vi "Kalman Calculation.vi"(4 "our_robots":bool=TRUE, 5 "u_k":T1, 6 "R":T1=[[0.1, 0.0, 0.0], [0.0, 0.1, 0.0], [0.0, 0.0, 0.1]], 7 "Use Observation":bool=TRUE, 8 "intervalo":dbl=1.0, 9 "Pk-1|k-1":T1, 10 "x_k-1|k-1":T1=[[0.0, 0.0, 0.0], [0.0, 0.0, 0.0], [0.0, 0.0, 0.0]], 11 "z_k":T1) -> (1 "Conf":dbl, 2 "Pk|k":T1, 3 "x_k|k":T1)   [LabVIEW 2017]
uses:
  <vilib>/Analysis/Matrix/Datatypes/RealMatrix.ctl
  <vilib>/Analysis/_algsub.llb/Real Matrix Norm.vi
  <vilib>/Analysis/Matrix/Numeric/Multiply/Multiply - RM,R.vi
  <vilib>/Analysis/Matrix/Numeric/Conversions/Array To Matrix - RA2.vi
  <vilib>/Analysis/Matrix/Numeric/Multiply/Multiply - RM,RM.vi
  <vilib>/Analysis/Matrix/Numeric/Add/Add - RM,RM.vi
  <vilib>/Analysis/baseanly.llb/Real Inverse Matrix.vi
  <vilib>/Analysis/Matrix/Numeric/Subtract/Subtract - RM,RM.vi
  <vilib>/Analysis/Matrix/NI_Matrix.lvlib
  <vilib>/Analysis/NI_AALBase.lvlib
  <vilib>/Analysis/NI_AALPro.lvlib
panel:
  out "In Range?":bool[][](array[boolean])
  in  "DesAccel_Max":dbl=10.0
  in  "zero":T1=[[0.0], [0.0], [0.0], [0.0], [0.0], [0.0]]
  in  "Accel_Max":dbl=10.0 format="%#_13g"
  out "appended array":T1
  out "K_k":T1
  out "Inverse Matrix":T1
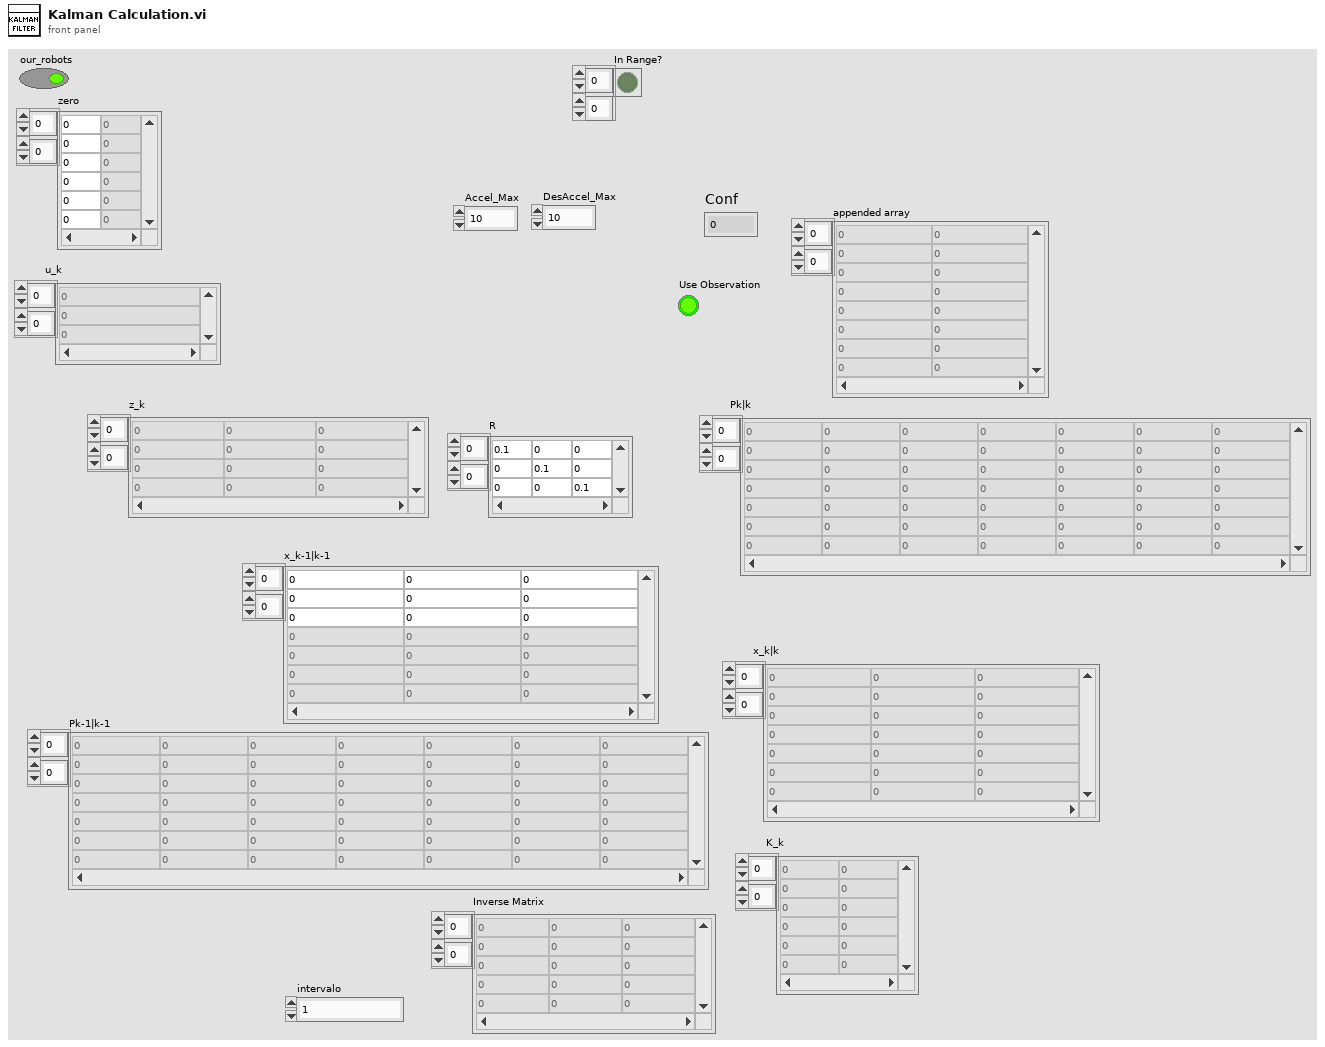
[diagram p1: front panel]
types:
  T1 = typedef "NI_Matrix.lvlib/RealMatrix.ctl" = dbl[][]
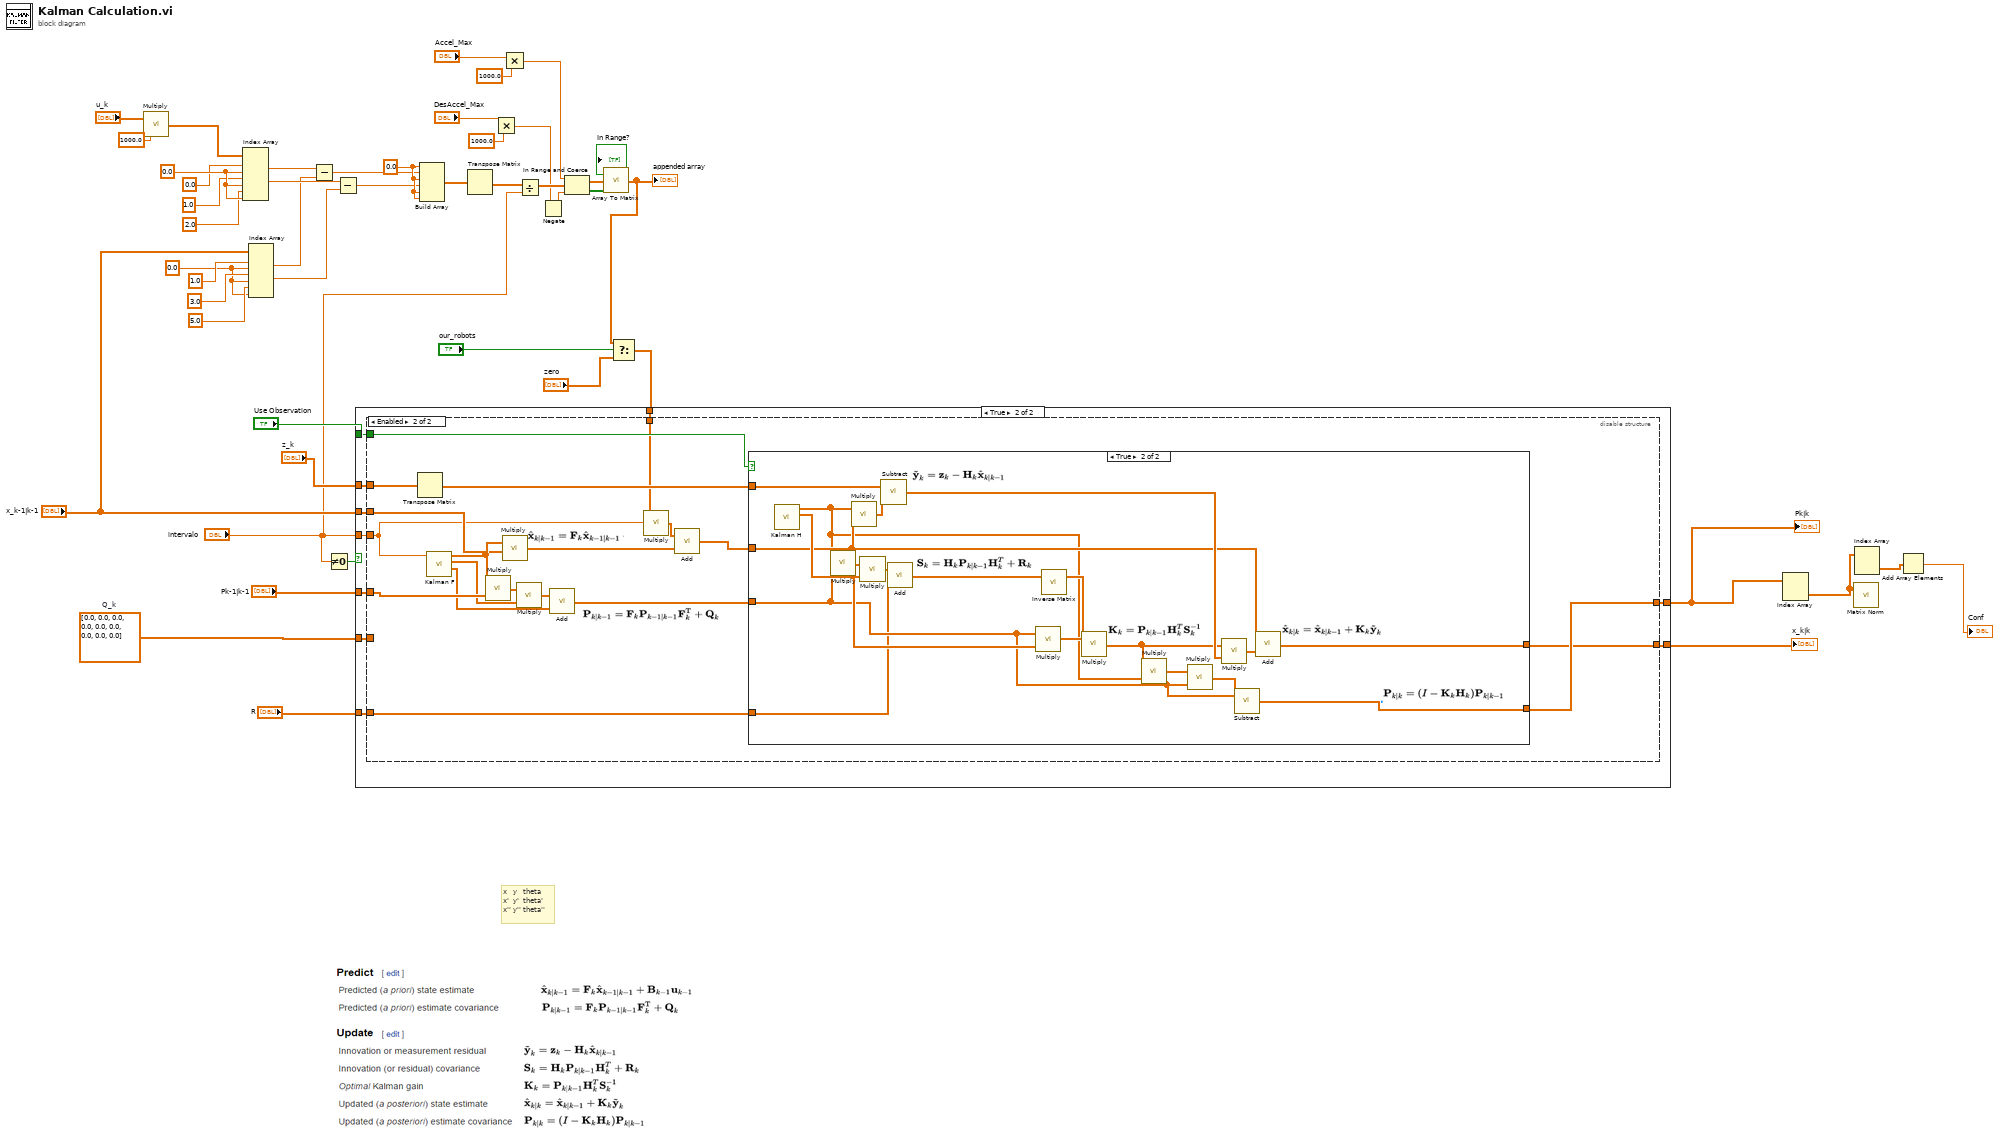
[diagram p0: block diagram]
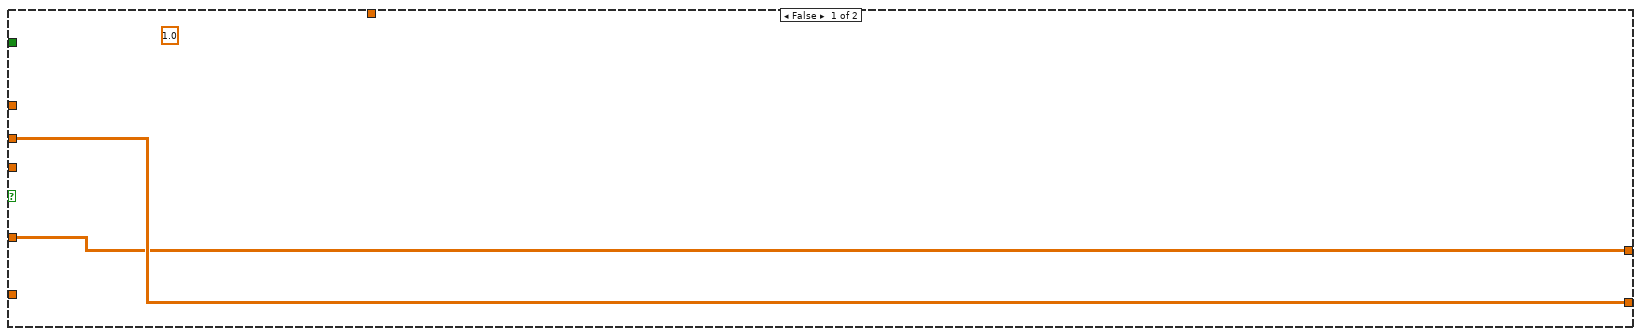
[diagram p2: hidden frame]
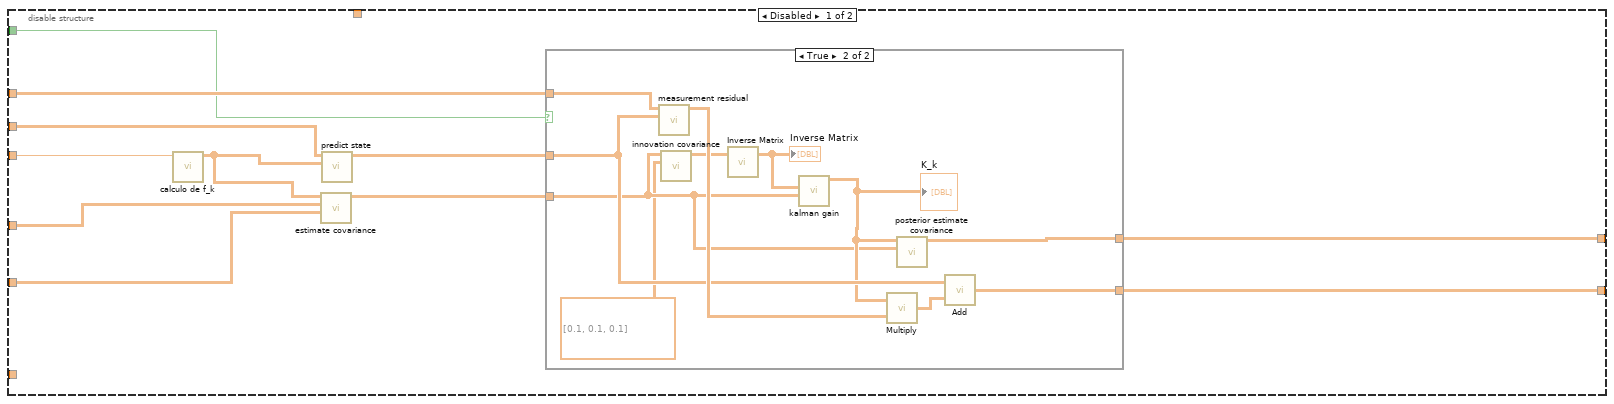
[diagram p3: hidden frame]
diagram:
  w27 = 0.0
  w35 = 0.0
  w36 = 0.0
  w44 = T1 [[0.0, 0.0, 0.0], [0.0, 0.0, 0.0], [0.0, 0.0, 0.0]]  # Q_k
  # "x   y   theta\nx'  y'  theta'\nx'' y'' theta''"
  n1 = call-poly <vilib>:"Multiply.vi"("Real Scalar c"=1000.0, "Real Matrix A"="u_k") -> ("A * c"=w8:T1)
  n2 = Index Array(array=w8, index (row) #1=0.0, index (col) #1=w36, index (row) #2=1.0, index (col) #2=w36, index (row) #3=2.0, index (col) #3=w36) -> (element #1=w22:dbl, element #2=w25:dbl)  [unwired: 1 out]
  n3 = Index Array(array="x_k-1|k-1", index (row) #1=1.0, index (col) #1=w27, index (row) #2=3.0, index (col) #2=w27, index (row) #3=5.0, index (col) #3=w27) -> (element #1=w23:dbl, element #2=w24:dbl)  [unwired: 1 out]
  n4 = Subtract(x=w22, y=w23) -> (x-y=w21:dbl)
  n5 = Not Equal To 0?(x="intervalo") -> (x != 0?=w45:bool)
  n6 = Subtract(x=w25, y=w24) -> (x-y=w20:dbl)
  n7 = Build Array(w35, w21, w35, w20, w35, w35) -> (w31:T1)
  n8 = Transpose Matrix(1:w31) -> (0:w19:T1)
  n9 = Multiply ("Multiply.vi")(x="DesAccel_Max", y=1000.0) -> (x*y=w1:dbl)
  n10 = Multiply ("Multiply.vi")(x="Accel_Max", y=1000.0) -> (x*y=w4:dbl)
  n11 = Divide(x=w19, y="intervalo") -> (x/y=w18:T1)
  n12 = Negate(x=w1) -> (-x=w11:dbl)
  n13 = In Range and Coerce(upper limit=w4, x=w18, lower limit=w11) -> (coerced(x)=w17:dbl[][], In Range?=→"In Range?":bool[][])
  n14 = call-poly <vilib>:"Array To Matrix.vi"("Real 2D Array"=w17) -> ("Real Matrix"=w15:T1)
  "appended array" <- w15
  n15 = Select(t=w15, s="our_robots", f="zero") -> (s? t:f=w13:T1)
  n16 = case shown="True" w45 {
    tunnel: "intervalo" -> [_ w59]
    tunnel: [w49 w58] -> w37
    tunnel: "Pk-1|k-1" -> [w48 w57]
    tunnel: "x_k-1|k-1" -> [w49 w55]
    tunnel: [w48 w56] -> w46
    tunnel: w44 -> [_ w54]
    tunnel: "z_k" -> [_ w53]
    tunnel: "Use Observation" -> [_ w52]
    tunnel: "R" -> [_ w51]
    tunnel: w13 -> [_ w50]
    frame False {
      (unwired) 1.0 ("intervalo")
    }
    frame True {
      n17 = disable-structure shown="Enabled" {
        disable-tunnel: w59 -> [w70 w84]
        disable-tunnel: [w67 w93] -> w58
        disable-tunnel: w57 -> [w66 w102]
        disable-tunnel: [w65 w94] -> w56
        disable-tunnel: w55 -> [w64 w91]
        disable-tunnel: w54 -> [w62 _]
        disable-tunnel: w53 -> [w61 w97]
        disable-tunnel: w52 -> [w60 w89]
        disable-tunnel: w51 -> [_ w90]
        disable-tunnel: w50 -> [_ w85]
        frame Disabled {
          n18 = call "calculo de f_k.vi"("iteração"=w70) -> ("F_k"=w63:T1)  [unwired: 10 in]
          n19 = call "estimate covariance.vi"("Q_k"=w62, "Pk-1|k-1"=w66, "F_k"=w63) -> ("Pk|k-1"=w68:T1)  [unwired: 8 in]
          n20 = call "predict state.vi"("F_k"=w63, "x_k-1|k-1"=w64) -> ("x_k|k-1"=w69:T1)  [unwired: 9 in]
          n21 = case shown="True" w60 {
            tunnel: [w72 w82] -> w67
            tunnel: w69 -> [w72 w80]
            tunnel: [w71 w77] -> w65
            tunnel: w68 -> [w71 w75]
            tunnel: w61 -> [_ w74]
            frame False {
            }
            frame True {
              n22 = call "measurement residual.vi"("x_k|k-1"=w80, "z_k"=w74) -> ("y~_k"=w81:T1)  [unwired: 9 in]
              n23 = call "innovation covariance.vi"("R"=T1 [[0.1, 0.1, 0.1]], "Pk|k-1"=w75) -> ("S_k"=w79:T1)  [unwired: 8 in, 1 out]
              n24 = call-poly <vilib>:"Inverse Matrix.vi"("Input Matrix"=w79) -> ("Inverse Matrix"=w78:T1)  [unwired: 1 in, 1 out]
              "Inverse Matrix" <- w78
              n25 = call "kalman gain.vi"("Pk|k-1"=w75, "S^-1"=w78) -> ("K_k"=w76:T1)  [unwired: 9 in]
              "K_k" <- w76
              n26 = call-poly <vilib>:"Multiply.vi"("Real Matrix B"=w81, "Real Matrix A"=w76) -> ("A * B"=w83:T1)
              n27 = call "posterior estimate covariance.vi"("Pk|k-1"=w75, "K_k"=w76) -> ("Pk|k"=w77:T1)  [unwired: 9 in]
              n28 = call-poly <vilib>:"Add.vi"("Real Matrix B"=w83, "Real Matrix A"=w80) -> ("A + B"=w82:T1)
            }
          }
        }
        frame Enabled {
          n29 = Transpose Matrix(1:w97) -> (0:w96:T1)
          n30 = call "Kalman F.vi"("intervalo"=w84) -> ("Q"=w98:T1, "F'"=w100:T1, "F"=w92:T1)  [unwired: 8 in]
          n31 = call-poly <vilib>:"Multiply.vi"("Real Matrix B"=w102, "Real Matrix A"=w92) -> ("A * B"=w101:T1)
          n32 = call-poly <vilib>:"Multiply.vi"("Real Matrix B"=w91, "Real Matrix A"=w92) -> ("A * B"=w88:T1)
          n33 = call-poly <vilib>:"Multiply.vi"("Real Matrix B"=w100, "Real Matrix A"=w101) -> ("A * B"=w99:T1)
          n34 = call-poly <vilib>:"Add.vi"("Real Matrix B"=w98, "Real Matrix A"=w99) -> ("A + B"=w95:T1)
          n35 = call-poly <vilib>:"Multiply.vi"("Real Scalar c"=w84, "Real Matrix A"=w85) -> ("A * c"=w86:T1)
          n36 = call-poly <vilib>:"Add.vi"("Real Matrix B"=w88, "Real Matrix A"=w86) -> ("A + B"=w87:T1)
          n37 = case shown="True" w89 {
            tunnel: w96 -> [_ w123]
            tunnel: w87 -> [w104 w113]
            tunnel: w95 -> [w103 w109]
            tunnel: [w103 w107] -> w94
            tunnel: [w104 w106] -> w93
            tunnel: w90 -> [_ w105]
            frame False {
            }
            frame True {
              n38 = call "Kalman H.vi"() -> ("H'"=w118:T1, "H"=w111:T1)  [unwired: 10 in]
              n39 = call-poly <vilib>:"Multiply.vi"("Real Matrix B"=w109, "Real Matrix A"=w111) -> ("A * B"=w121:T1)
              n40 = call-poly <vilib>:"Multiply.vi"("Real Matrix B"=w113, "Real Matrix A"=w111) -> ("A * B"=w122:T1)
              n41 = call-poly <vilib>:"Multiply.vi"("Real Matrix B"=w118, "Real Matrix A"=w121) -> ("A * B"=w120:T1)
              n42 = call-poly <vilib>:"Subtract.vi"("Real Matrix B"=w122, "Real Matrix A"=w123) -> ("A - B"=w115:T1)
              n43 = call-poly <vilib>:"Add.vi"("Real Matrix B"=w105, "Real Matrix A"=w120) -> ("A + B"=w119:T1)
              n44 = call-poly <vilib>:"Multiply.vi"("Real Matrix B"=w118, "Real Matrix A"=w109) -> ("A * B"=w117:T1)
              n45 = call-poly <vilib>:"Inverse Matrix.vi"("Input Matrix"=w119) -> ("Inverse Matrix"=w116:T1)  [unwired: 1 in, 1 out]
              n46 = call-poly <vilib>:"Multiply.vi"("Real Matrix B"=w116, "Real Matrix A"=w117) -> ("A * B"=w112:T1)
              n47 = call-poly <vilib>:"Multiply.vi"("Real Matrix B"=w111, "Real Matrix A"=w112) -> ("A * B"=w110:T1)
              n48 = call-poly <vilib>:"Multiply.vi"("Real Matrix B"=w109, "Real Matrix A"=w110) -> ("A * B"=w108:T1)
              n49 = call-poly <vilib>:"Multiply.vi"("Real Matrix B"=w115, "Real Matrix A"=w112) -> ("A * B"=w114:T1)
              n50 = call-poly <vilib>:"Subtract.vi"("Real Matrix B"=w108, "Real Matrix A"=w109) -> ("A - B"=w107:T1)
              n51 = call-poly <vilib>:"Add.vi"("Real Matrix B"=w114, "Real Matrix A"=w113) -> ("A + B"=w106:T1)
            }
          }
        }
      }
    }
  }
  "Pk|k" <- w46
  "x_k|k" <- w37
  n52 = Index Array(array=w46) -> (element=w40:T1)  [unwired: 2 in]
  n53 = call-poly <vilib>:"Matrix Norm.vi"("Input Matrix"=w40) -> ()  [unwired: 1 in, 2 out]
  n54 = Index Array(array=w40) -> (element=w39:T1)  [unwired: 2 in]
  n55 = Add Array Elements(numeric array=w39) -> (sum=→"Conf":dbl)
